vi "Write TCS string.vi"(8 "error in (no error)":errorcluster, 10 "TCS string":string, 11 "Telemetry in":refnum<class "Telemetry.lvclass">) -> (0 "error out":errorcluster, 3 "Telemetry out":refnum<class "Telemetry.lvclass">)   [LabVIEW 2018, in "Telemetry.lvclass"]
uses:
  Telemetry.lvclass
  Telemetry.lvclass/Telemetry.ctl
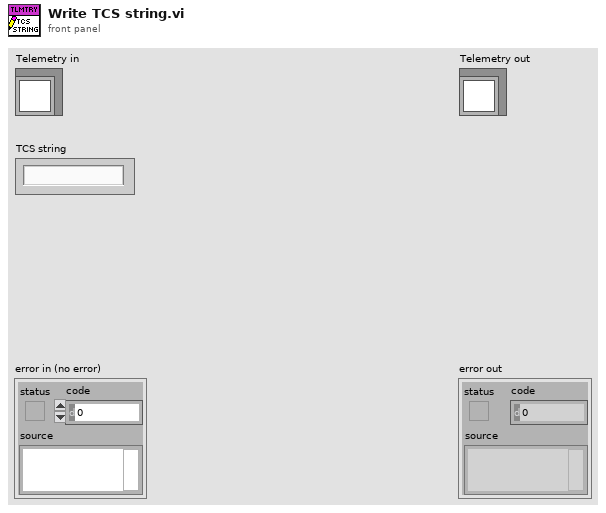
[diagram p1: front panel]
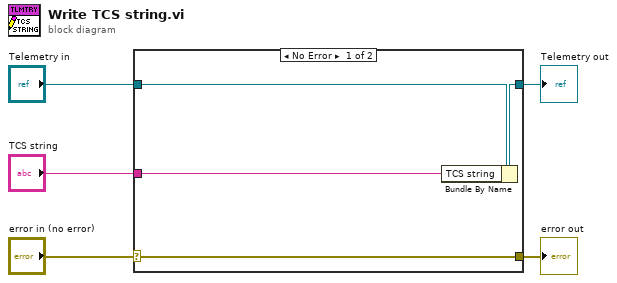
[diagram p0: block diagram]
diagram:
  n1 = case shown="No Error" "error in (no error)" {
    selector: "error in (no error)" -> [w9 w10]
    tunnel: [w9 w10] -> w4
    tunnel: [w7 w11] -> w2
    tunnel: "Telemetry in" -> [w8 w11]
    tunnel: "TCS string" -> [w6 _]
    frame No Error {
      n2 = Bundle By Name(cluster=w8, "TCS string"=w6) -> (w7:refnum<class "Telemetry.lvclass">)
    }
    frame Error {
    }
  }
  "error out" <- w4
  "Telemetry out" <- w2
